vi "RecipeFile_List.vi"() -> ()   [LabVIEW 2014]
panel:
  in  "Data_Ctl_List":u16(ring) items=["None", "Config_RFSA_IQ_Acq", "Config_RFSA_Spectrum_Acq", "Config_RFSA_Vertical", "Config_RFSG"]
  in  "RFSA_State":u16(ring) items=["RFSA_Init", "RFSA_Init_Servo", "Config_RFSA_AcqType_Vertical", "Config_RFSA_IQ_Acq", "Config_RFSA_Spectrum_Acq", "Config_RFSA_Trigger", "RFSA_Initiate", "RFSA_Fetch_IQ", "RFSA_Acq_Read_Spectrum", "RFSA_Acq_Read_IQ", "RFSA_Stop", "RFSA_Close", "Wait_Cmd", "Send_Cmd", "Exit"]
  in  "State List of RFSA":string[](array[string])=["===== Device Init =====", "RFSA_Init", "RFSA_Init_Servo", "===== Configure =====", "Config_RFSA_AcqType_Vertical", "Config_RFSA_IQ_Acq", "Config_RFSA_Spectrum_Acq", "Config_RFSA_Trigger", "===== Acquisition =====", "RFSA_Initiate", "RFSA_Fetch_IQ", "RFSA_Acq_Read_Spectrum", "RFSA_Acq_Read_IQ", "===== Sesion Stop&Close =====", "RFSA_Stop", "RFSA_Close", "===== Operation =====", "Wait_Cmd", "Send_Cmd", "Exit"]
  in  "State List of RFSG":string[](array[string])=[" ===== Device Init =====", "RFSG_Init", "RFSG_Init_Servo", "===== Configure =====", "Config_ScriptWfm", "Config_Freq_Power_ExtGain", "Config_RFSG_Mode_CW", "Config_RFSG_Mode_Script", "===== Generation =====", "RFSG_Write_Script", "RFSG_Initiate", "===== Session Stop&Close =====", "RFSG_Stop", "RFSG_Close", "===== Operation =====", "Wait_Cmd", "Send_Cmd", "Exit"]
  in  "RFSG_State":u16(ring) items=["RFSG_Init", "RFSG_Init_Servo", "Config_ScriptWfm", "Config_Freq_Power_ExtGain", "Config_RFSG_Mode_CW", "Config_RFSG_Mode_Script", "RFSG_Write_Script", "RFSG_Initiate", "RFSG_Stop", "RFSG_Close", "Wait_Cmd", "Send_Cmd", "Exit"]
  # "[ Recipe Maker ]"
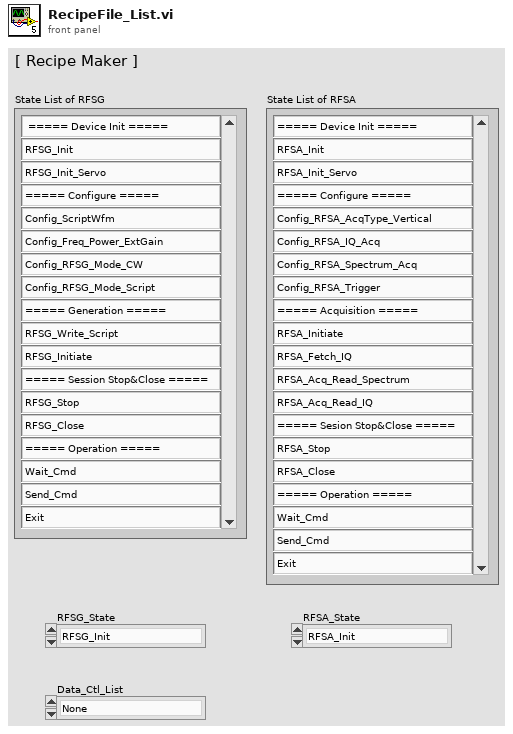
[diagram p1: front panel]
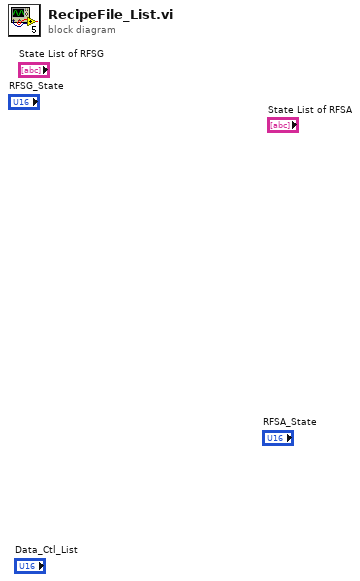
[diagram p0: block diagram]
diagram:
